vi "Memory.Pointer.Copy All.Safe.vi"(8 "error in (no error)":errorcluster, 10 "dst pointer in":refnum<class "Memory.Pointer.lvclass">, 11 "src pointer in":refnum<class "Memory.Pointer.lvclass">) -> (0 "error out":errorcluster, 2 "dst pointer out":refnum<class "Memory.Pointer.lvclass">, 3 "src pointer out":refnum<class "Memory.Pointer.lvclass">)   [LabVIEW 2016, in "Memory.lvlib" / "Memory.Pointer.lvclass"]
doc: "Copies all of the data from the memory address specified by <b>src pointer</b> to the memory address specified by <b>dst pointer</b>.\n\n<b>Note:</b> This VI is <b>safe</b>.\n\nSafe means that this function evaluates that the size parameter of <b>dst pointer</b> is greater than or equal to the size of <b>src pointer</b> to ensure that the destination memory location is an appropriate size before copying data from source to destination. Reading/writing more data to a pointer than it has allocated can corrupt or crash LabVIEW."
uses:
  Memory.Pointer.lvclass
  Memory.Pointer.lvclass/Memory.Pointer.ctl
  Memory.Pointer.Copy.Unsafe.vi
  Memory.Pointer.Parameter Check.Subset.vi
  Memory.Pointer.Parameter Check.Null Pointer.vi
  Memory.Pointer.Get Address.vi
  Memory.Pointer.Errors.vi
  Memory.Pointer.Errors.Out of Bounds.vi
  Memory.Pointer.Errors.Null Pointer.vi
  Submodules/SEH/Source/VIs/Static Error Handling.Source Buffer.Write.String.vi
  Memory.Pointer.Errors.Write Pointer Size.vi
  Memory.Pointer.Errors.Create Error.vi
  Submodules/SEH/Source/VIs/Static Error Handling.Source Buffer.Write.Numeric.Scalar.Base10.vi
  Submodules/SEH/Source/VIs/Static Error Handling.Source Buffer.Write.Numeric.Scalar.Base10 (U64).vi
  Submodules/SEH/Source/VIs/Static Error Handling.Error Cluster Constant.vi
  Submodules/SEH/Source/VIs/Static Error Handling.Error Cluster Constant (256B).vi
  Submodules/SEH/Source/VIs/Static Error Handling.Parameters.Status.Set.vi
  Submodules/SEH/Source/VIs/Static Error Handling.Parameters.Code.Set.vi
  Submodules/SEH/Source/VIs/Static Error Handling.Parameters.VI Source.Set.vi
  Constants/Memory.Constants.vi
  Constants/Memory.Constants.Library Name.vi
  Memory.Pointer.Errors.Get Info.vi
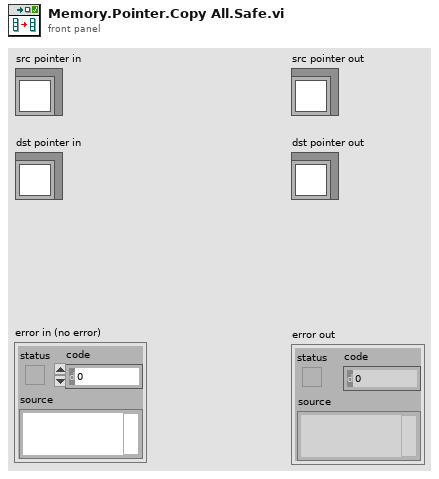
[diagram p1: front panel]
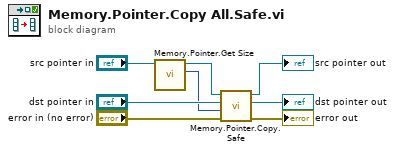
[diagram p0: block diagram]
diagram:
  n1 = call "Memory.Pointer.Get Size.vi"("Pointer in"="src pointer in") -> ("size"=w5:u64, "Pointer out"=w7:refnum<class "Memory.Pointer.lvclass">)  [unwired: 8 in, 1 out]
  n2 = call "Memory.Pointer.Copy.Safe.vi"("error in (no error)"="error in (no error)", "bytes to copy"=w5, "dst pointer in"="dst pointer in", "src pointer in"=w7) -> ("error out"=→"error out":errorcluster, "dst pointer out"=→"dst pointer out":refnum<class "Memory.Pointer.lvclass">, "src pointer out"=→"src pointer out":refnum<class "Memory.Pointer.lvclass">)  [unwired: 4 in, 1 out]
